vi "Find All Subsequences.vi"(11 "JO4M":u16[](array[numeric])) -> (3 "All Subarrays Out":T1[](array[typedef]))   [LabVIEW 2013, in "GA.lvclass"]
uses:
  GA.lvclass
  Controls/Subsequence.ctl
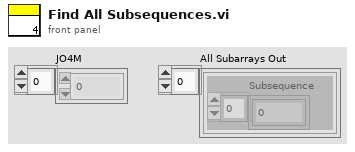
[diagram p1: front panel]
types:
  T1 = typedef "Subsequence.ctl" = cluster{"Subsequence":i32[]}
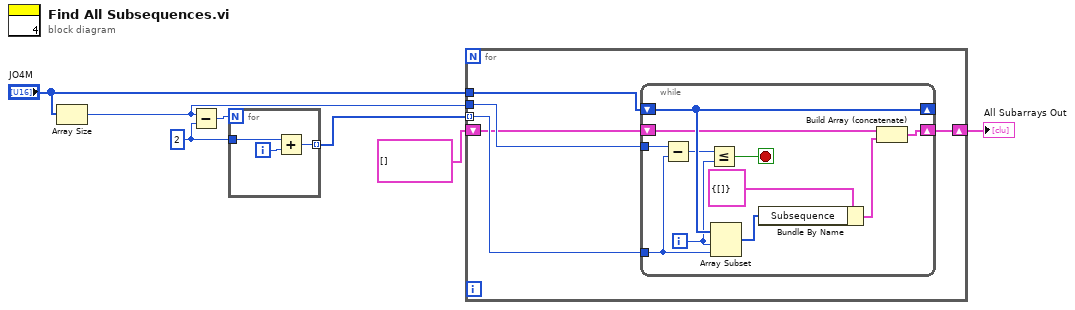
[diagram p0: block diagram]
diagram:
  w4 = 2 ("y")
  n1 = Array Size(array="JO4M") -> (size(s)=w2:i32)
  n2 = Subtract(x=w2, y=w4) -> (x-y=w5:i32)
  n3 = for {
    N: w5 -> [_]
    tunnel: w4 -> [w9]
    tunnel: [w8] -> w3 mode=indexing
    i -> [w10]
    n4 = Add(x=w9, y=w10) -> (x+y=w8:i32)
  }
  n5 = for {
    tunnel: "JO4M" -> [w15]
    tunnel: w3 -> [w14] mode=indexing
    tunnel: w2 -> [w13]
    shift-right: [w11] -> w7
    shift-left: T1[] [] -> [w12]
    n6 = while {
      shift-right: [w20] -> _
      shift-left: w15 -> [w20]
      tunnel: w14 -> [w23]
      tunnel: w13 -> [w26]
      shift-right: [w16] -> w11
      shift-left: w12 -> [w17]
      i -> [w18]
      stop <- w25 stop-if-true
      n7 = Subtract(x=w26, y=w23) -> (x-y=w19:i32)
      n8 = Less Or Equal?(x=w19, y=w18) -> (x <= y?=w25:bool)
      n9 = Array Subset(array=w20, index=w18, length=w23) -> (w22:u16[])
      n10 = Bundle By Name(cluster=T1 {"Subsequence"=[]}, "Subsequence"=w22) -> (w21:T1)
      n11 = Build Array (concatenate)(w17, w21) -> (w16:T1[])
    }
  }
  "All Subarrays Out" <- w7
